vi "four_function_calculator.vi"() -> ()   [LabVIEW 2020]
panel:
  out "DIVISION":dbl
  out "MULTIPLICATION":dbl
  out "SUBTRACTION":dbl
  out "ADDITION":dbl
  in  "Y":dbl
  in  "X":dbl
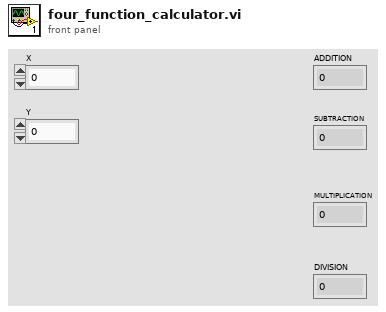
[diagram p1: front panel]
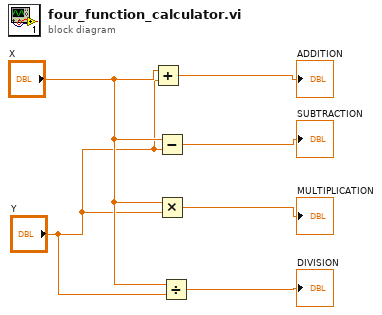
[diagram p0: block diagram]
diagram:
  n1 = Add(x="X", y="Y") -> (x+y=→"ADDITION":dbl)
  n2 = Subtract(x="X", y="Y") -> (x-y=→"SUBTRACTION":dbl)
  n3 = Multiply(x="X", y="Y") -> (x*y=→"MULTIPLICATION":dbl)
  n4 = Divide(x="X", y="Y") -> (x/y=→"DIVISION":dbl)
